vi "process error.vi"(10 "Error Object":refnum<class "Error.lvclass">, 11 "Error Interface in":refnum<class "Error Interface.lvclass">) -> ()   [LabVIEW 2020, in "Error Interface.lvlib" / "Error Interface.lvclass"]
uses:
  Error Interface.lvclass
  Error/Error.lvclass
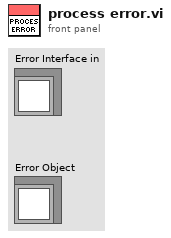
[diagram p1: front panel]
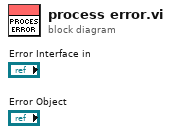
[diagram p0: block diagram]
diagram:
